vi "Compute P(x).vi"(6 "timeout (1000 ms)":i32=1000, 8 "error in (no error)":errorcluster, 10 "x":dbl, 11 "PolyA in":refnum<class "PolyA.lvclass">) -> (0 "error out":errorcluster, 2 "P(x)":dbl, 3 "PolyA out":refnum<class "PolyA.lvclass">)   [LabVIEW 2014, in "PolyA.lvclass"]
uses:
  PolyA.lvclass
  Query Payload -- cluster.ctl
  PolyA.lvclass/PolyA.ctl
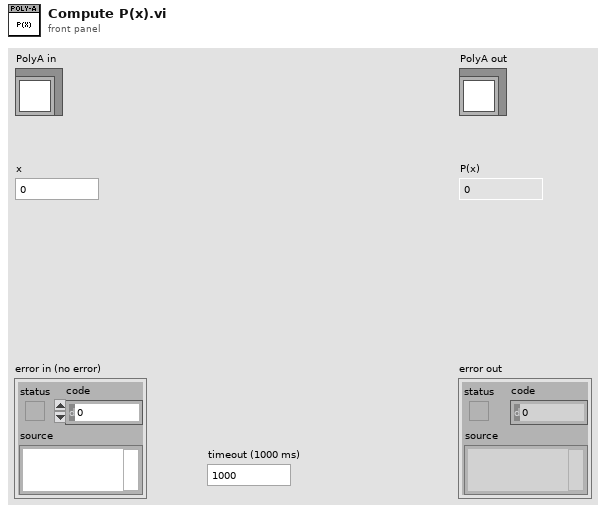
[diagram p1: front panel]
types:
  T1 = typedef "PolyA.lvclass/Query Payload -- cluster.ctl" = cluster{"value":dbl, "notifier":refnum<notifier>}
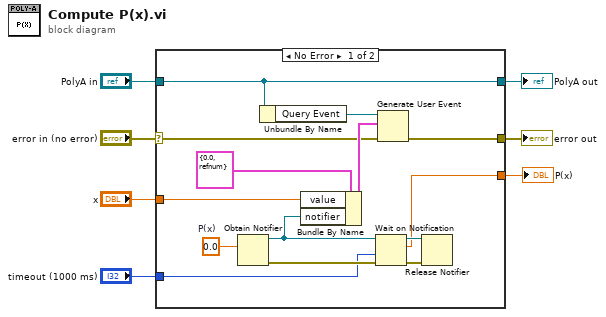
[diagram p0: block diagram]
diagram:
  n1 = case shown="No Error" "error in (no error)" {
    selector: "error in (no error)" -> [w9 w23]
    tunnel: [w8 w23] -> w6
    tunnel: [w15 w22] -> w4
    tunnel: "PolyA in" -> [w15 w22]
    tunnel: "timeout (1000 ms)" -> [w19 _]
    tunnel: [w16 _] -> w2
    tunnel: "x" -> [w12 _]
    frame No Error {
      w21 = 0.0  # P(x)
      n2 = Obtain Notifier(notification data type=w21) -> (notifier out=w11:refnum<notifier>, error out=w20:errorcluster)  [unwired: 3 in, 1 out]
      n3 = Unbundle By Name(w15) -> ("Query Event"=w14:refnum<user-event>)
      n4 = Bundle By Name(cluster=T1 {"value"=0.0, "notifier"=refnum} ("Query Payload"), "value"=w12, "notifier"=w11) -> (w10:T1)
      n5 = Wait on Notification(notifier=w11, timeout in ms (-1)=w19, error in (no error)=w20) -> (notifier out=w18:refnum<notifier>, notification=w16:dbl, error out=w17:errorcluster)  [unwired: 1 in, 1 out]
      n6 = Generate User Event(user event=w14, event data cluster=w10, error in=w9) -> (error out=w8:errorcluster)  [unwired: 1 in, 1 out]
      n7 = Release Notifier(notifier=w18, error in (no error)=w17) -> ()  [unwired: 1 in, 3 out]
    }
    frame Error {
    }
  }
  "error out" <- w6
  "PolyA out" <- w4
  "P(x)" <- w2
